vi "Load Framework.vi"(8 "error in (no error)":errorcluster, 10 "Test Framework Type":T1) -> (0 "error out":errorcluster, 2 "Test Framework Instance":refnum<class "Test Framework.lvclass">)   [LabVIEW 2017, in "Framework.lvlib" / "Test Framework Factory.lvclass"]
uses:
  Test Framework Factory.lvclass
  Test Framework/Test Framework.lvclass
  Test Framework.ctl
  LVUnit Test Framework/LVUnit Test Framework.lvclass
  C:/Users/pasca/Projects/Home/lvunit/Framework/Test Framework/Test Framework.lvclass
  Framework.lvlib
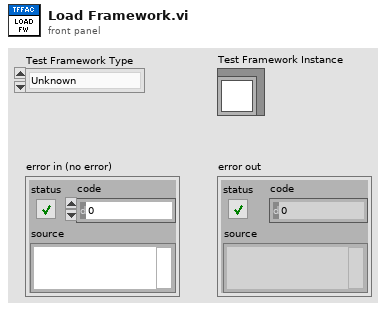
[diagram p1: front panel]
types:
  T1 = typedef "Framework.lvlib/Test Framework.ctl" = enum16{"Unknown", "LVUnit", "Caraya"}
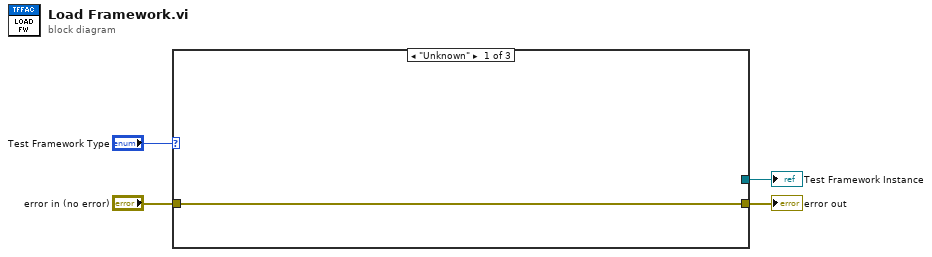
[diagram p0: block diagram]
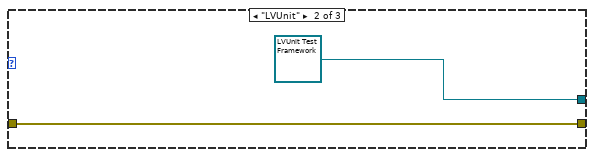
[diagram p2: hidden frame]
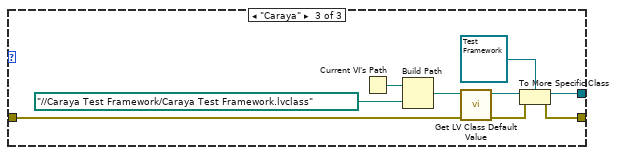
[diagram p3: hidden frame]
diagram:
  n1 = case shown="\"Unknown\"" "Test Framework Type" {
    tunnel: "error in (no error)" -> [w5 w7 w11]
    tunnel: [w5 w7 w9] -> w3
    tunnel: [_ refnum<class "LVUnit Test Framework.lvclass"> refnum ("Framework.lvlib:LVUnit Test Framework.lvclass") w8] -> w2
    frame "Unknown" {
    }
    frame "LVUnit" {
    }
    frame "Caraya" {
      n2 = Current VI's Path() -> (path=w15:path)
      n3 = Build Path(base path=w15, name or relative path=path "../../Caraya Test Framework/Caraya Test Framework.lvclass") -> (appended path=w14:path)
      n4 = call <vilib>:"Get LV Class Default Value.vi"("error in (no error)"=w11, "class path"=w14) -> ("error out"=w10:errorcluster, "object"=w13:refnum<class>)  [unwired: 8 in]
      n5 = To More Specific Class(target class=refnum<class "Test Framework.lvclass"> refnum ("Framework.lvlib:Test Framework.lvclass"), reference=w13, error in=w10) -> (specific class reference=w8:refnum<class "Test Framework.lvclass">, error out=w9:errorcluster)
    }
  }
  "error out" <- w3
  "Test Framework Instance" <- w2
